vi "lab 8.vi"() -> ()   [LabVIEW 2021]
uses:
  <vilib>/MakerHub/LINX/Public/Utilities/Open Serial.vi
  <vilib>/MakerHub/LINX/Public/Sensors/Motion/Servo/Servo Open One Channel.vi
  <vilib>/MakerHub/LINX/Public/Sensors/Motion/Servo/Servo Set Pulse Width One Channel.vi
  <vilib>/MakerHub/LINX/Public/Sensors/Motion/Servo/Servo Close One Channel.vi
  <vilib>/MakerHub/LINX/LMH-LINX.lvlib
  <vilib>/MakerHub/LINX/Public/Sensors/Motion/Servo/Servo.lvlib
panel:
  in  "stop":bool
  out "Angle":dbl(graph)
  out "Angle":dbl
  in  "Knob":u16(knob) scale=500.0..2500.0
  in  "Servo Channel":u8
  in  "Serial Port":refnum<visa-resource-name>="N/A"
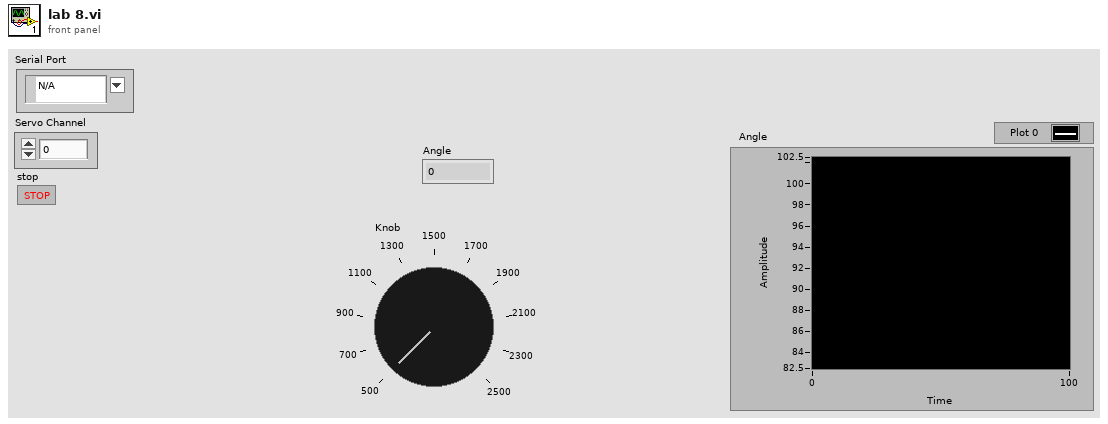
[diagram p1: front panel]
types:
  T1 = typedef "LMH-LINX.lvlib/LINX Ref.ctl" = cluster{"IO":T2, "Interface":T3, "LINX Device Config":T4}
  T2 = typedef "LMH-LINX.lvlib/Platform.ctl" = enum16{"Remote", "Local"}
  T3 = typedef "LMH-LINX.lvlib/Interface.ctl" = enum16{"Serial", "TCP"}
  T4 = typedef "LMH-LINX.lvlib/Device.lvlib/LINX Device Config.ctl" = cluster{"Interface":T3, "COM Port":refnum<visa-resource-name>, "TCP Configuration":T5, "Device Family":u8, "Device ID":u8, "Device Name":string, "TCP Ref":refnum<k5>, "Channels":T6}
  T5 = typedef "LMH-LINX.lvlib/Device.lvlib/TCP Config.ctl" = cluster{"IP Address":string, "Port":u16}
  T6 = typedef "LMH-LINX.lvlib/Channels.ctl" = cluster{"DI":u8[], "DO":u8[], "AI":u8[], "AO":u8[], "PWM":u8[], "QE":u8[], "UART":u8[], "I2C 2":u8[], "SPI":u8[], "CAN":u8[], "Servo":u8[], "AI Ref (V)":dbl, "AI Resolution (Bits)":u8, "AO Ref (V)":dbl, "AO Resolution (Bits)":u8}
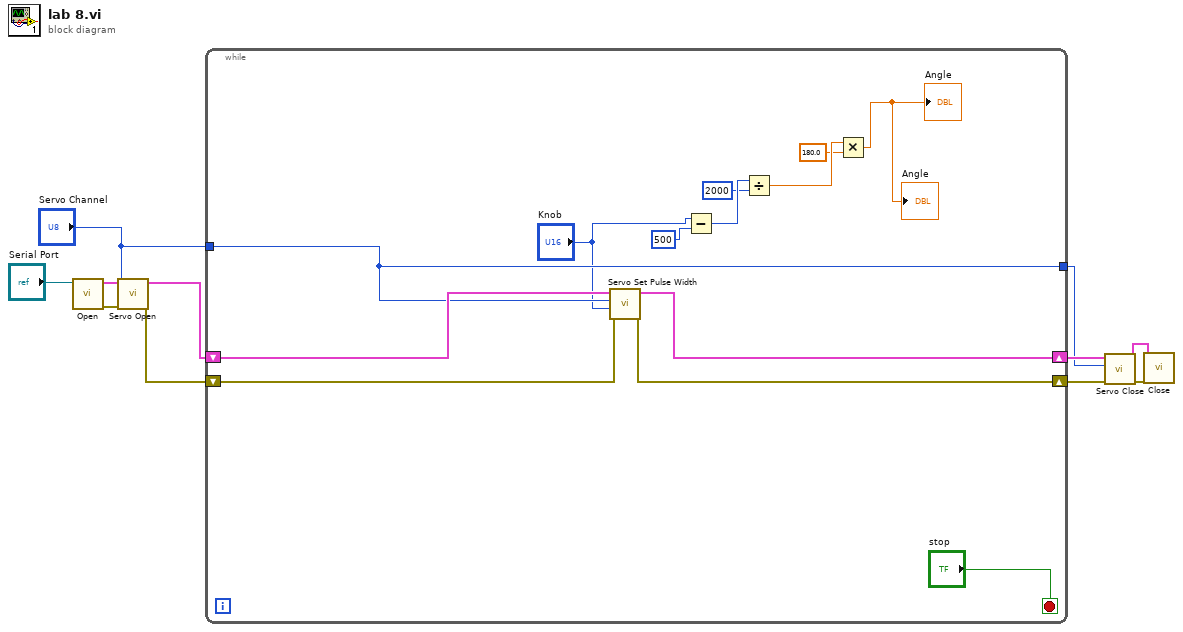
[diagram p0: block diagram]
diagram:
  n1 = call-poly <vilib>:"Open.vi"("Serial Port"="Serial Port") -> ("Error Out"=w10:errorcluster, "LINX Resource"=w9:T1)  [unwired: 8 in, 1 out]
  n2 = call-poly <vilib>:"Servo Open.vi"("Error In"=w10, "Servo Channel"="Servo Channel", "LINX Resource"=w9) -> ("Error Out"=w6:errorcluster, "LINX Resource"=w7:T1)  [unwired: 7 in]
  n3 = while {
    tunnel: "Servo Channel" -> [w20]
    tunnel: [w20] -> w1
    shift-right: [w22] -> w3
    shift-left: w7 -> [w24]
    shift-right: [w21] -> w2
    shift-left: w6 -> [w23]
    stop <- "stop" stop-if-true
    n4 = call-poly <vilib>:"Servo Set Pulse Width.vi"("Error In"=w23, "Pulse Width (uS)"="Knob", "Servo Channel"=w20, "LINX Resource"=w24) -> ("Error Out"=w21:errorcluster, "LINX Resource"=w22:T1)  [unwired: 6 in]
    n5 = Subtract(x="Knob", y=u16 500) -> (x-y=w17:u16)
    n6 = Divide(x=w17, y=u16 2000) -> (x/y=w15:dbl)
    n7 = Multiply(x=w15, y=180.0) -> (x*y=→"Angle" →"Angle":dbl)
  }
  n8 = call-poly <vilib>:"Servo Close.vi"("Error In"=w2, "Servo Channel"=w1, "LINX Resource"=w3) -> ("Error Out"=w5:errorcluster, "LINX Resource"=w4:T1)  [unwired: 7 in]
  n9 = call <vilib>:"Close.vi"("Error In"=w5, "LINX Resource"=w4) -> ()  [unwired: 9 in, 1 out]
